vi "Core.vi"(8 "error in (no error)":errorcluster, 11 "Module in":refnum<class "Module.lvclass">) -> ()   [LabVIEW 2020, in "Module.lvlib" / "Module.lvclass"]
uses:
  Module.lvclass
  <vilib>/Utility/error.llb/Error Cluster From Error Code.vi
  <vilib>/ErrorRing/Error Ring.xnode
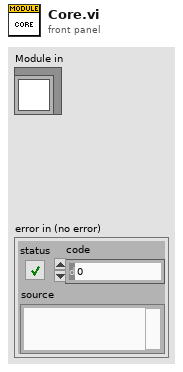
[diagram p1: front panel]
types:
  T1 = enum32{"Invalid", "Standard", "Closed", "Hidden", "Minimized", "Maximized"}
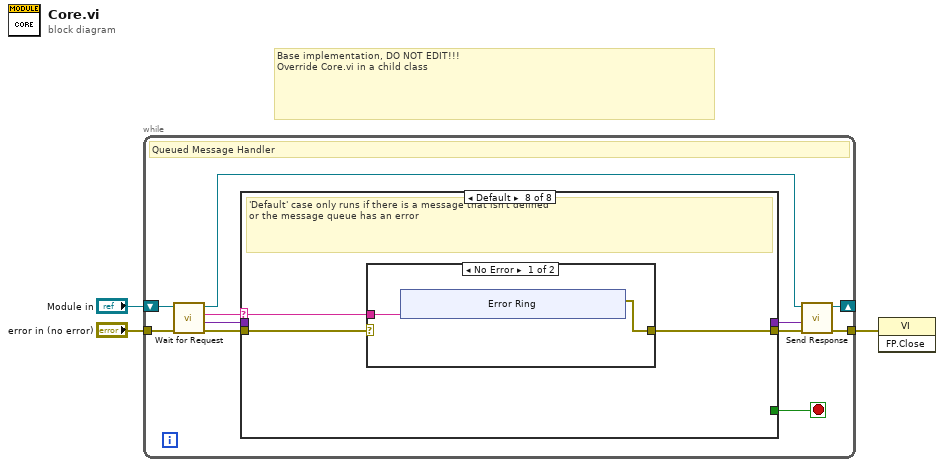
[diagram p0: block diagram]
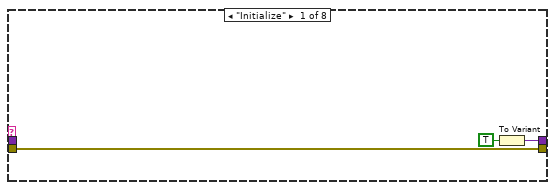
[diagram p2: hidden frame]
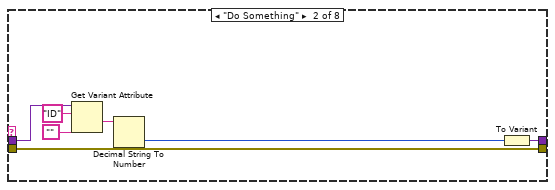
[diagram p3: hidden frame]
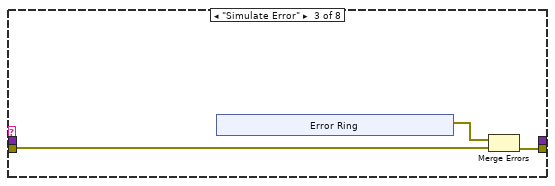
[diagram p4: hidden frame]
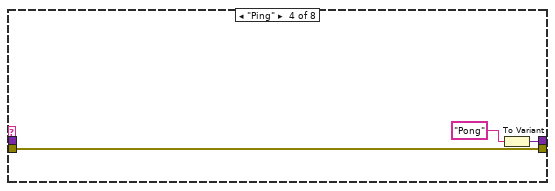
[diagram p5: hidden frame]
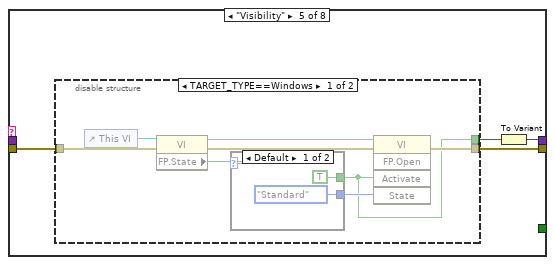
[diagram p6: hidden frame]
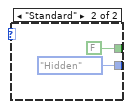
[diagram p7: hidden frame]
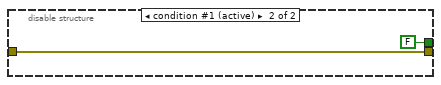
[diagram p8: hidden frame]
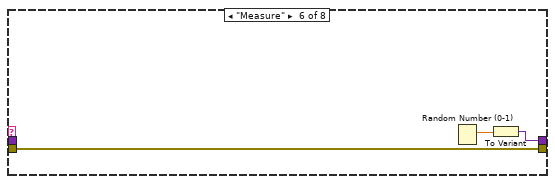
[diagram p9: hidden frame]
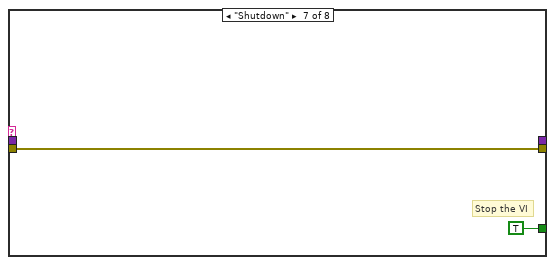
[diagram p10: hidden frame]
diagram:
  # "Base implementation, DO NOT EDIT!!!\nOverride Core.vi in a child class"
  n1 = while {
    shift-right: [w14] -> _
    shift-left: "Module in" -> [w10]
    tunnel: "error in (no error)" -> [w8]
    tunnel: [w11] -> w1
    stop <- w9 stop-if-true
    # "Queued Message Handler"
    n2 = call "Wait for Request.vi"("error in"=w8, "Module in"=w10) -> ("error out"=w7:errorcluster, "Data"=w6:variant, "Message"=w4:string, "Module out"=w5:refnum<class "Module.lvclass">)  [unwired: 6 in]
    n3 = case shown="Default" w4 {
      selector: w4 -> [_ _ _ _ _ _ _ w60]
      tunnel: w7 -> [w15 w20 w26 w35 w39 w56 w57 w61]
      tunnel: [_ _ _ _ _ _ TRUE _] -> w9
      tunnel: w6 -> [_ w21 _ _ _ _ _ _]
      tunnel: [w17 w19 _ w34 w37 w55 _ _] -> w13
      tunnel: [w15 w20 w27 w35 w38 w56 w57 w59] -> w12
      frame "Initialize" {
        n4 = To Variant(anything=TRUE) -> (Variant=w17:variant)
      }
      frame "Do Something" {
        n5 = Get Variant Attribute(Variant=w21, name="ID", default value (empty Variant)="") -> (value=w22:string)  [unwired: 1 in, 3 out]
        n6 = Decimal String To Number(string=w22) -> (number=w18:i32)  [unwired: 2 in, 1 out]
        n7 = To Variant(anything=w18) -> (Variant=w19:variant)
      }
      frame "Simulate Error" {
        n8 = xnode "Error Ring"() -> ("error out"=w25:errorcluster)
        n9 = Merge Errors(w25, w26) -> (w27:errorcluster)
      }
      frame "Ping" {
        n10 = To Variant(anything="Pong") -> (Variant=w34:variant)
      }
      frame "Visibility" {
        n11 = disable-structure shown="TARGET_TYPE==Windows" {
          disable-tunnel: w39 -> [w47 w53]
          disable-tunnel: [w42 w53] -> w38
          disable-tunnel: [w41 FALSE ("Activate?")] -> w36
          frame condition #0 {
            n12 = control-ref of="This VI"() -> (w40:refnum<vi>)
            n13 = property class="VI"(reference=w40, error in=w47) -> (reference out=w45:refnum<vi>, error out=w46:errorcluster, "FP.State"=w44:T1)
            n14 = case shown="Default" w44 {
              tunnel: [T1."Standard" ("State") T1."Hidden" ("State")] -> w43
              tunnel: [TRUE ("Activate?") FALSE ("Activate?")] -> w41
              frame Default {
              }
              frame "Standard" {
              }
            }
            n15 = invoke class="VI" method="FP.Open"(reference=w45, error in=w46, "Activate"=w41, "State"=w43) -> (error out=w42:errorcluster)  [unwired: 1 in, 4 out]
          }
          frame condition #1 (active) {
          }
        }
        n16 = To Variant(anything=w36) -> (Variant=w37:variant)
      }
      frame "Measure" {
        n17 = Random Number (0-1)() -> (number: 0 to 1=w54:dbl)
        n18 = To Variant(anything=w54) -> (Variant=w55:variant)
      }
      frame "Shutdown" {
        # "Stop the VI"
      }
      frame Default {
        # "'Default' case only runs if there is a message that isn't defined\nor the message queue has an error"
        n19 = case shown="No Error" w61 {
          selector: w61 -> [_ w71]
          tunnel: w60 -> [w63 _]
          tunnel: [w62 w71] -> w59
          frame No Error {
            n20 = xnode ("Error Ring")("parameter 0"=w63) -> ("error out"=w62:errorcluster)
          }
          frame Error {
          }
        }
      }
    }
    n21 = call "Send Response.vi"("error in"=w12, "Response"=w13, "Module in"=w5) -> ("error out"=w11:errorcluster, "Module out"=w14:refnum<class "Module.lvclass">)  [unwired: 7 in]
  }
  n22 = invoke class="VI" method="FP.Close"(error in=w1) -> ()  [unwired: 2 in, 3 out]
